vi "Read ItemsList.vi"(8 "error in (no error)":errorcluster, 11 "Msg_Error.lvclass in":refnum<class "ListSelection.lvclass">) -> (0 "error out":errorcluster, 2 "Items List":string[](array[string]), 3 "Msg_Error.lvclass out":refnum<class "ListSelection.lvclass">)   [LabVIEW 2012, in "ListSelection.lvlib" / "ListSelection.lvclass"]
uses:
  ListSelection.lvclass
  ListSelection.lvclass/ListSelection.ctl
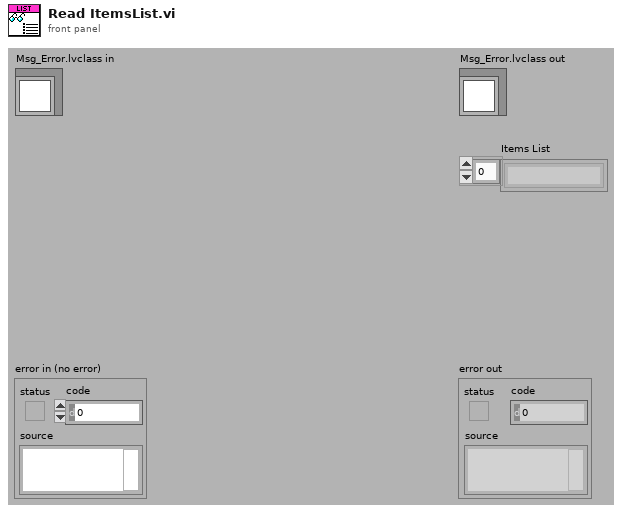
[diagram p1: front panel]
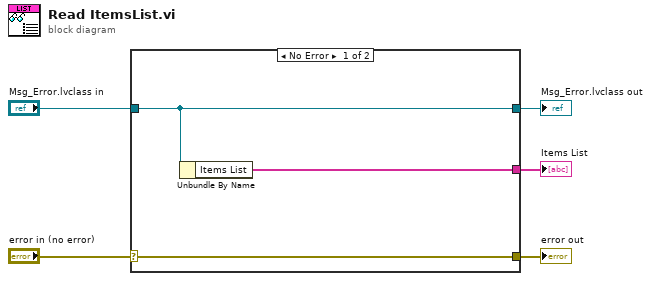
[diagram p0: block diagram]
diagram:
  n1 = case shown="No Error" "error in (no error)" {
    selector: "error in (no error)" -> [w8 w9]
    tunnel: [w8 w9] -> w4
    tunnel: [w7 w10] -> w2
    tunnel: "Msg_Error.lvclass in" -> [w7 w10]
    tunnel: [w6 _] -> w1
    frame No Error {
      n2 = Unbundle By Name(w7) -> ("Items List"=w6:string[])
    }
    frame Error {
    }
  }
  "error out" <- w4
  "Msg_Error.lvclass out" <- w2
  "Items List" <- w1
